vi "B_WriteAttribute.vi"(8 "error in (no error)":errorcluster, 11 "reference in":refnum<class "BaseTemplate_4x4x4.lvclass">) -> (0 "error out":errorcluster, 3 "reference out":refnum<class "BaseTemplate_4x4x4.lvclass">)   [LabVIEW 2020]
uses:
  <resource>/Framework/Providers/Open_GDS/ClassProviders/Provider_EndevoGOOP300/Templates/BaseTemplate_4x4x4/BaseTemplate_4x4x4.lvclass
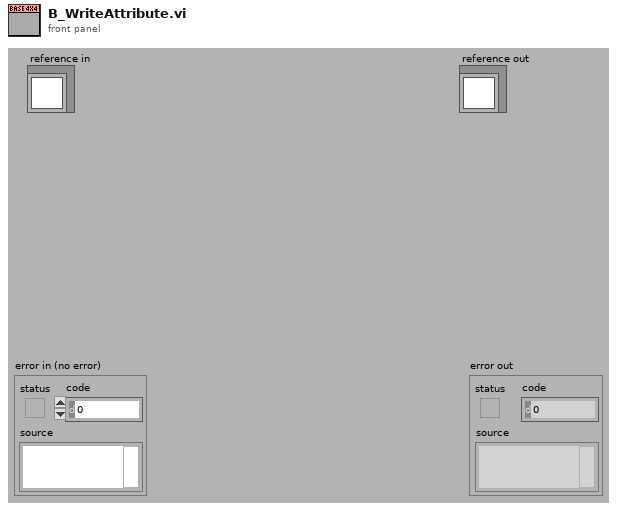
[diagram p1: front panel]
types:
  T1 = typedef "BaseTemplate_4x4x4.lvclass/ObjectAttributes.ctl" = cluster{"Attribute1":dbl}
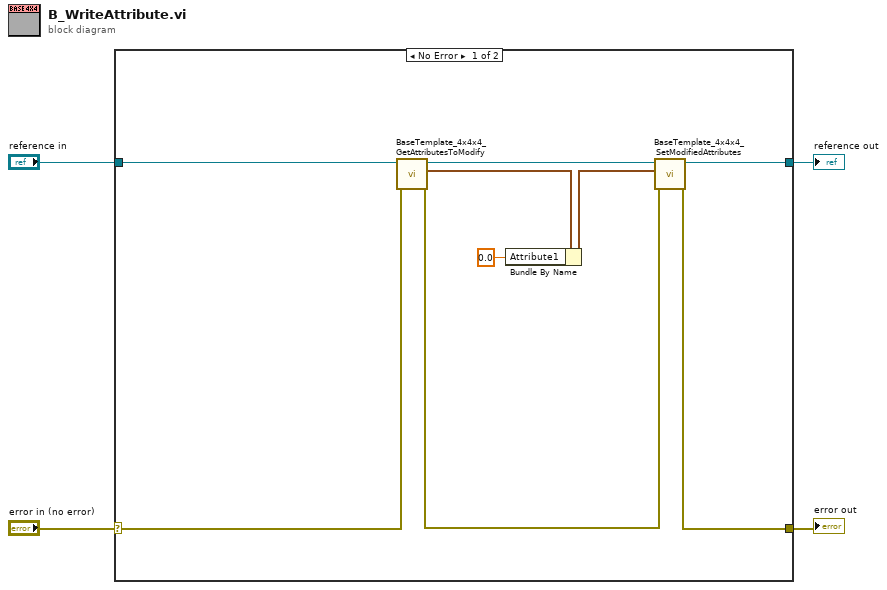
[diagram p0: block diagram]
diagram:
  n1 = case shown="No Error" "error in (no error)" {
    selector: "error in (no error)" -> [w8 w15]
    tunnel: [w10 w15] -> w3
    tunnel: [w7 w14] -> w1
    tunnel: "reference in" -> [w9 w14]
    frame No Error {
      n2 = call <resource>:"BaseTemplate_4x4x4_GetAttributesToModify.vi"("error in (no error)"=w8, "reference in"=w9) -> ("error out"=w5:errorcluster, "Attributes"=w13:T1, "reference out"=w11:refnum<class "BaseTemplate_4x4x4.lvclass">)  [unwired: 6 in, 1 out]
      n3 = Bundle By Name(cluster=w13, "Attribute1"=0.0) -> (w12:T1)
      n4 = call <resource>:"BaseTemplate_4x4x4_SetModifiedAttributes.vi"("error in (no error)"=w5, "Attributes"=w12, "reference in"=w11) -> ("error out"=w10:errorcluster, "reference out"=w7:refnum<class "BaseTemplate_4x4x4.lvclass">)  [unwired: 7 in]
    }
    frame Error {
    }
  }
  "error out" <- w3
  "reference out" <- w1
